vi "Search Line Scan Point.vi"(11 "Station Action in":refnum<class "Station Action.lvclass">) -> (0 "TrayIndex":cluster{"IndexX":i32, "IndexY":i32}, 1 "End":cluster{"X":sgl, "Y":sgl}, 2 "Start":cluster{"X":sgl, "Y":sgl}, 3 "None":bool)   [LabVIEW 2019]
uses:
  Class/Main Process Class/MPC_AutoPaste/Station Class/Station Action.lvclass
panel:
  out "IndexY":i32
  out "IndexX":i32
  out "Station Action out":refnum<class "Station Action.lvclass">
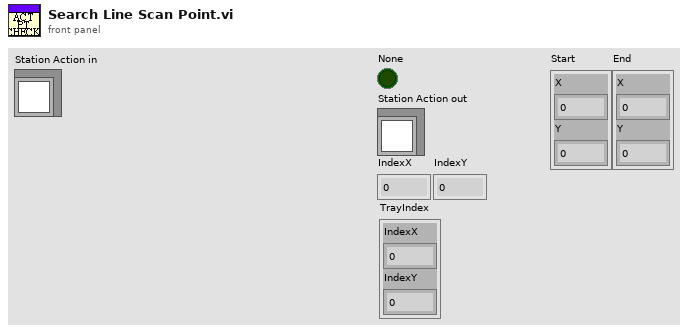
[diagram p1: front panel]
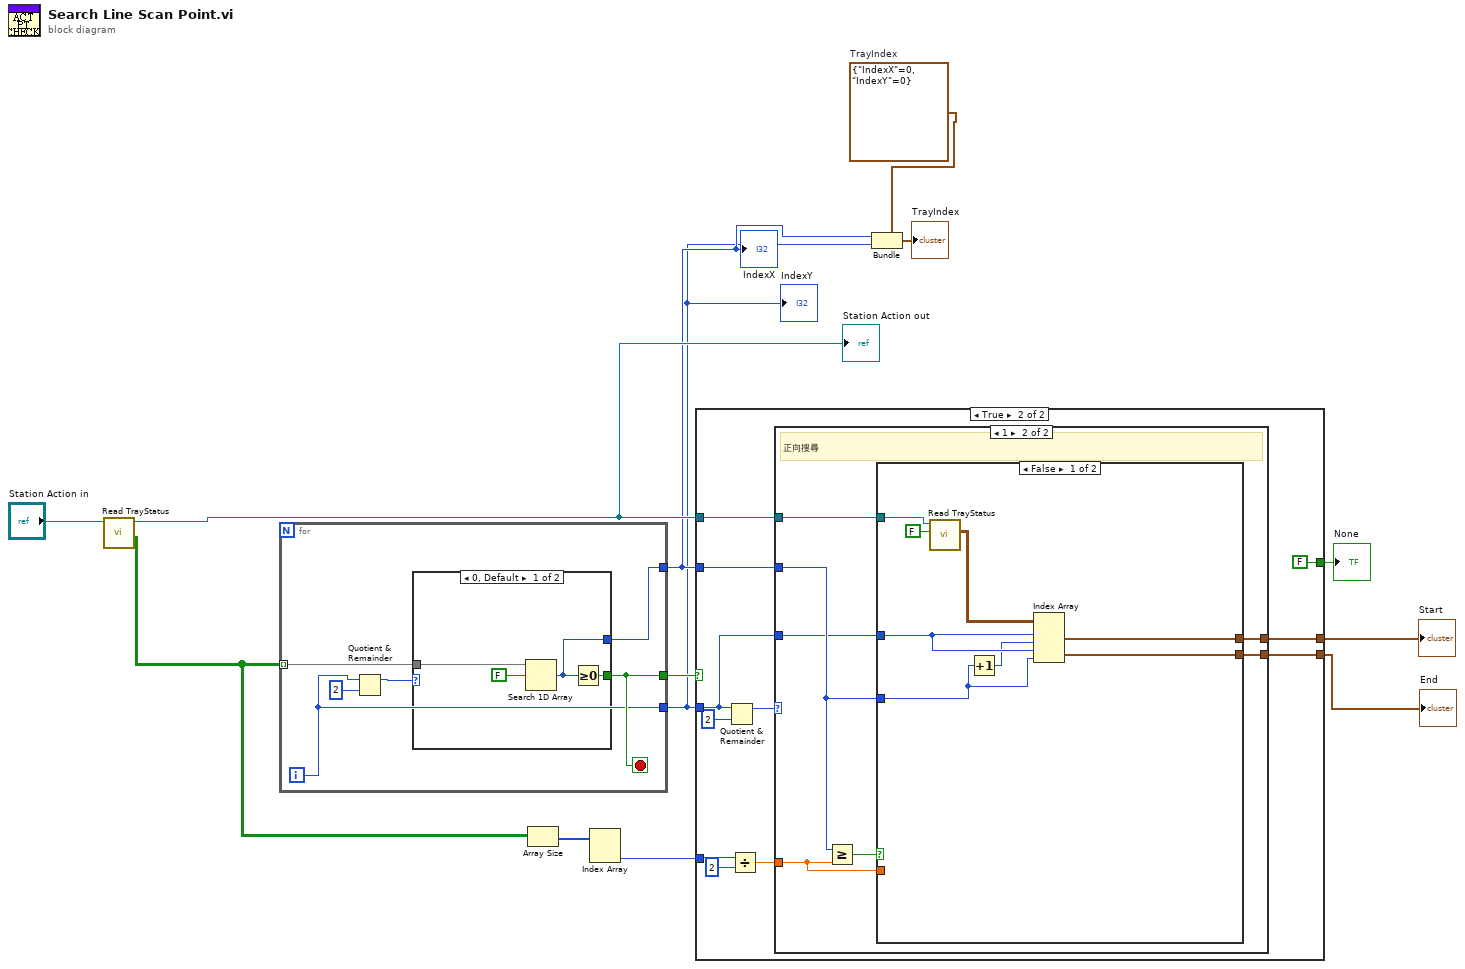
[diagram p0: block diagram]
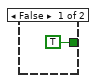
[diagram p2: hidden frame]
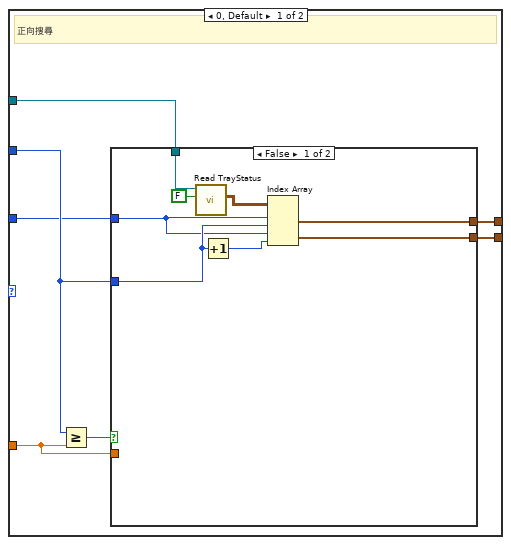
[diagram p3: hidden frame]
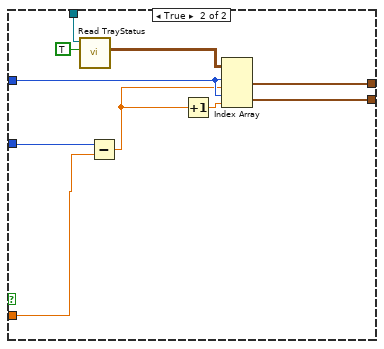
[diagram p4: hidden frame]
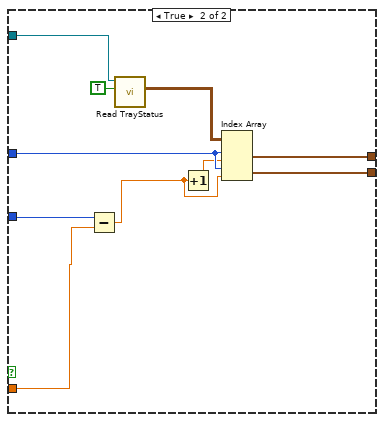
[diagram p5: hidden frame]
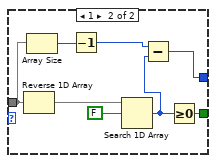
[diagram p6: hidden frame]
diagram:
  w2 = cluster{"IndexX":i32, "IndexY":i32} {"IndexX"=0, "IndexY"=0}  # TrayIndex
  n1 = call-dynamic "Read TrayStatus.vi"("Station Action in"="Station Action in") -> ("Arr_TrayST"=w7:bool[][], "Station Action out"=w6:refnum<class "Station Action.lvclass">)  [unwired: 7 in, 2 out]
  "Station Action out" <- w6
  n2 = for {
    tunnel: w7 -> [w19] mode=indexing
    tunnel: [w18] -> w13
    tunnel: [w15] -> w3
    tunnel: [w17] -> w4
    i -> [w15]
    stop <- w18 stop-if-true
    n3 = Quotient & Remainder(x=w15, y=2) -> (x-y*floor(x/y)=w14:i32)  [unwired: 1 out]
    n4 = case shown="0, Default" w14 {
      tunnel: w19 -> [w23 w28]
      tunnel: [w21 w30] -> w18
      tunnel: [w20 w25] -> w17
      frame 0, Default {
        n5 = Search 1D Array(1D array=w23, element=FALSE) -> (index of element=w20:i32)  [unwired: 1 in]
        n6 = Greater Or Equal To 0?(x=w20) -> (x >= 0?=w21:bool)
      }
      frame 1 {
        n7 = Reverse 1D Array(array=w28) -> (reversed array=w29:bool[])
        n8 = Array Size(array=w28) -> (size(s)=w27:i32)
        n9 = Decrement(x=w27) -> (x-1=w24:i32)
        n10 = Search 1D Array(1D array=w29, element=FALSE) -> (index of element=w26:i32)  [unwired: 1 in]
        n11 = Subtract(x=w24, y=w26) -> (x-y=w25:i32)
        n12 = Greater Or Equal To 0?(x=w26) -> (x >= 0?=w30:bool)
      }
    }
  }
  "IndexX" <- w4
  "IndexY" <- w3
  n13 = Array Size(array=w7) -> (size(s)=w12:i32[])
  n14 = Index Array(array=w12) -> (element #2=w11:i32)  [unwired: 2 in, 1 out]
  n15 = case shown="True" w13 {
    tunnel: w3 -> [_ w35]
    tunnel: w4 -> [_ w41]
    tunnel: w11 -> [_ w40]
    tunnel: [_ w37] -> w10
    tunnel: [_ w36] -> w9
    tunnel: [TRUE FALSE] -> w8
    tunnel: w6 -> [_ w33]
    frame False {
    }
    frame True {
      n16 = Quotient & Remainder(x=w35, y=2) -> (x-y*floor(x/y)=w42:i32)  [unwired: 1 out]
      n17 = Divide(x=w40, y=2) -> (x/y=w38:dbl)
      n18 = case shown="1" w42 {
        tunnel: w41 -> [w46 w71]
        tunnel: w38 -> [w47 w72]
        tunnel: [w49 w74] -> w37
        tunnel: [w48 w73] -> w36
        tunnel: w35 -> [w45 w70]
        tunnel: w33 -> [w44 w69]
        frame 0, Default {
          # "正向搜尋"
          n19 = Greater Or Equal?(x=w46, y=w47) -> (x >= y?=w50:bool)
          n20 = case shown="False" w50 {
            tunnel: w46 -> [w57 w65]
            tunnel: [w56 w68] -> w49
            tunnel: [w55 w67] -> w48
            tunnel: w47 -> [_ w64]
            tunnel: w45 -> [w54 w66]
            tunnel: w44 -> [w52 w59]
            frame False {
              n21 = call-dynamic "Read TrayStatus.vi"("F1/T2"=FALSE, "Station Action in"=w52) -> ("Arr_Tray"=w53:cluster{"X":sgl, "Y":sgl}[][])  [unwired: 6 in, 3 out]
              n22 = Increment(x=w57) -> (x+1=w58:i32)
              n23 = Index Array(array=w53, index (row) #1=w54, index (col) #1=w57, index (row) #2=w54, index (col) #2=w58) -> (element #1=w56:cluster{"X":sgl, "Y":sgl}, element #2=w55:cluster{"X":sgl, "Y":sgl})
            }
            frame True {
              n24 = call-dynamic "Read TrayStatus.vi"("F1/T2"=TRUE, "Station Action in"=w59) -> ("Arr_Tray"=w60:cluster{"X":sgl, "Y":sgl}[][])  [unwired: 6 in, 3 out]
              n25 = Subtract(x=w65, y=w64) -> (x-y=w63:dbl)
              n26 = Increment(x=w63) -> (x+1=w62:dbl)
              n27 = Index Array(array=w60, index (row) #1=w66, index (col) #1=w63, index (row) #2=w66, index (col) #2=w62) -> (element #1=w68:cluster{"X":sgl, "Y":sgl}, element #2=w67:cluster{"X":sgl, "Y":sgl})
            }
          }
        }
        frame 1 {
          # "正向搜尋"
          n28 = Greater Or Equal?(x=w71, y=w72) -> (x >= y?=w75:bool)
          n29 = case shown="False" w75 {
            tunnel: w71 -> [w79 w90]
            tunnel: [w83 w93] -> w74
            tunnel: [w82 w92] -> w73
            tunnel: w72 -> [_ w89]
            tunnel: w70 -> [w81 w91]
            tunnel: w69 -> [w78 w86]
            frame False {
              n30 = call-dynamic "Read TrayStatus.vi"("F1/T2"=FALSE, "Station Action in"=w78) -> ("Arr_Tray"=w76:cluster{"X":sgl, "Y":sgl}[][])  [unwired: 6 in, 3 out]
              n31 = Increment(x=w79) -> (x+1=w80:i32)
              n32 = Index Array(array=w76, index (row) #1=w81, index (col) #1=w80, index (row) #2=w81, index (col) #2=w79) -> (element #1=w83:cluster{"X":sgl, "Y":sgl}, element #2=w82:cluster{"X":sgl, "Y":sgl})
            }
            frame True {
              n33 = Subtract(x=w90, y=w89) -> (x-y=w87:dbl)
              n34 = call-dynamic "Read TrayStatus.vi"("F1/T2"=TRUE, "Station Action in"=w86) -> ("Arr_Tray"=w84:cluster{"X":sgl, "Y":sgl}[][])  [unwired: 6 in, 3 out]
              n35 = Increment(x=w87) -> (x+1=w88:dbl)
              n36 = Index Array(array=w84, index (row) #1=w91, index (col) #1=w88, index (row) #2=w91, index (col) #2=w87) -> (element #1=w93:cluster{"X":sgl, "Y":sgl}, element #2=w92:cluster{"X":sgl, "Y":sgl})
            }
          }
        }
      }
    }
  }
  "Start" <- w10
  "End" <- w9
  "None" <- w8
  n37 = Bundle(cluster=w2, "IndexX"=w4, "IndexY"=w3) -> (→"TrayIndex":cluster{"IndexX":i32, "IndexY":i32})
